vi "ChangeWhileMeasuring.vi"(8 "error in (no error)":errorcluster, 11 "PacificPowerSource in":refnum<class "PacificPowerSource.lvclass">) -> (0 "error out":errorcluster, 1 "MeasurementSettings":bool, 2 "OutputOrLoadValue":bool, 3 "PacificPowerSource out":refnum<class "PacificPowerSource.lvclass">)   [LabVIEW 2018, in "AcPwrPlugins.lvlib" / "PacificPowerSource.lvclass"]
doc: "This VI checks if the instrument is capable of send new instrument setting while the instruments is currently acquiring measurements."
uses:
  PacificPowerSource.lvclass
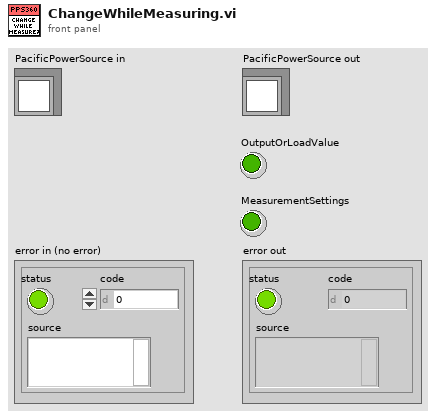
[diagram p1: front panel]
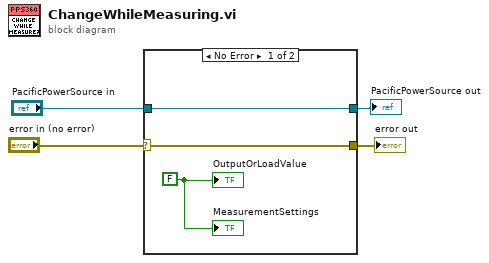
[diagram p0: block diagram]
diagram:
  n1 = case shown="No Error" "error in (no error)" {
    selector: "error in (no error)" -> [w6 w9]
    tunnel: [w6 w9] -> w2
    tunnel: [w7 w8] -> w1
    tunnel: "PacificPowerSource in" -> [w7 w8]
    frame No Error {
      w5 = FALSE ("OutputOrLoadState")
      "MeasurementSettings" <- w5
      "OutputOrLoadValue" <- w5
    }
    frame Error {
    }
  }
  "error out" <- w2
  "PacificPowerSource out" <- w1
